vi "ATS_InputControl.vi"(7 "ID":i32, 9 "InputControl":T1 {"Range" items=["20mV", "40mV", "50mV", "80mV", "100mV", "200mV", "400mV", "500mV", "800mV", "1 V", "1.25 V", "2 V", "4 V", "5 V", "8 V", "10 V", "16 V", "20 V", "40 V", "HiFi"]}, 10 "Channel":T6, 11 "HandleIn":u32) -> (0 "Return Code":u32, 1 "OutputControl":T1 {"Range" items=["20mV", "40mV", "50mV", "80mV", "100mV", "200mV", "400mV", "500mV", "800mV", "1 V", "1.25 V", "2 V", "4 V", "5 V", "8 V", "10 V", "16 V", "20 V", "40 V", "HiFi"]}, 2 "Range_Value":dbl format="%.3f", 3 "HandleOut":u32)   [LabVIEW 2010]
doc: "_____AlazarTech, Scope_____\n\nConfigure an input channel for acquisition.\n\n- Channel\n- Coupling\n- Range\n- Impedance\n- Bandwidth (if applicable)"
uses:
  ATS_ctl/InputCtrl.ctl
  ATS_ctl/Coupling.ctl
  ATS_ctl/Range.ctl
  ATS_ctl/Impedance.ctl
  ATS_ctl/Bandwidth.ctl
  ATS_ctl/ATS_Channel.ctl
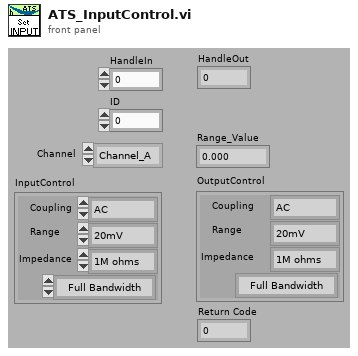
[diagram p1: front panel]
types:
  T1 = typedef "InputCtrl.ctl" = cluster{"Coupling":T2, "Range":T3, "Impedance":T4, "Bandwidth":T5}
  T2 = typedef "Coupling.ctl" = enum16{"AC", "DC"}
  T3 = typedef "Range.ctl" = u32
  T4 = typedef "Impedance.ctl" = enum16{"1M ohms", "50 ohms"}
  T5 = typedef "Bandwidth.ctl" = enum16{"Full Bandwidth", "Reduce Bandwidth"}
  T6 = typedef "ATS_Channel.ctl" = enum16{"Channel_A", "Channel_B", "Channel_C", "Channel_D"}
  T7 = typedef "ATS_Card_Spec.ctl" = cluster{"Name":string, "Rate":string[], "Range":string[], "RangeLim(50)":u32, "Bandwidth":bool}
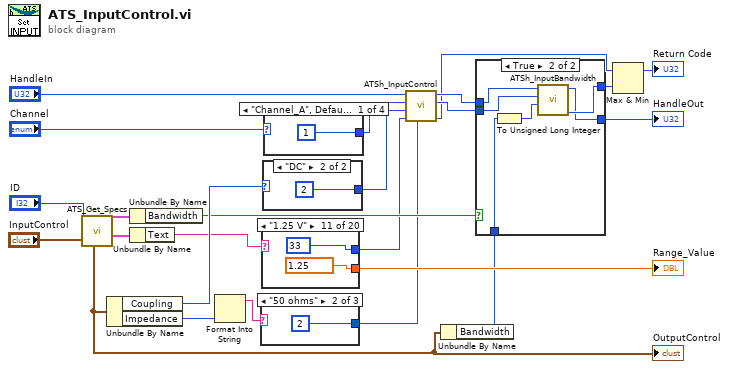
[diagram p0: block diagram]
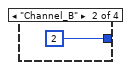
[diagram p2: hidden frame]
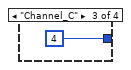
[diagram p3: hidden frame]
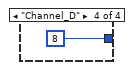
[diagram p4: hidden frame]
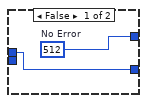
[diagram p5: hidden frame]
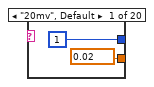
[diagram p6: hidden frame]
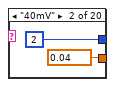
[diagram p7: hidden frame]
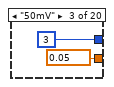
[diagram p8: hidden frame]
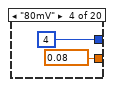
[diagram p9: hidden frame]
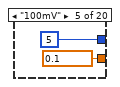
[diagram p10: hidden frame]
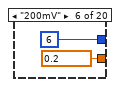
[diagram p11: hidden frame]
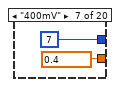
[diagram p12: hidden frame]
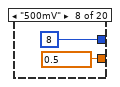
[diagram p13: hidden frame]
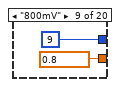
[diagram p14: hidden frame]
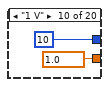
[diagram p15: hidden frame]
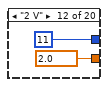
[diagram p16: hidden frame]
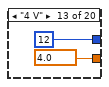
[diagram p17: hidden frame]
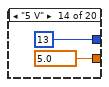
[diagram p18: hidden frame]
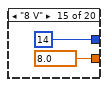
[diagram p19: hidden frame]
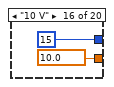
[diagram p20: hidden frame]
diagram:
  n1 = call "ATS_Get_Specs.vi"("InputControl"="InputControl", "ID"="ID") -> ("Range_Out"=w20:cluster{"Text":string, "Range":u32}, "Card_Spec"=w19:T7, "OutputControl"=w10:T1)  [unwired: 5 in, 2 out]
  "OutputControl" <- w10
  n2 = Unbundle By Name(w10) -> ("Coupling"=w24:T2, "Impedance"=w14:T4)
  n3 = Unbundle By Name(w19) -> ("Bandwidth"=w18:bool)
  n4 = Unbundle By Name(w20) -> ("Text"=w22:string)
  n5 = Format Into String(w14) -> (resulting string=w13:string)  [unwired: 3 in, 1 out]
  n6 = case shown="\"50 ohms\"" w13 {
    tunnel: [u32 1 ("Channel") u32 2 ("Channel") u32 8 ("Channel")] -> w5
    frame "1M ohms", Default {
    }
    frame "50 ohms" {
    }
    frame "300 ohms" {
    }
  }
  n7 = case shown="\"1.25 V\"" w22 {
    tunnel: [u32 1 ("Channel") u32 2 ("Channel") u32 3 ("Channel") u32 4 ("Channel") u32 5 ("Channel") u32 6 ("Channel") u32 7 ("Channel") u32 8 ("Channel") u32 9 ("Channel") u32 10 ("Channel") u32 33 ("Channel") u32 11 ("Channel") u32 12 ("Channel") u32 13 ("Channel") u32 14 ("Channel") u32 15 ("Channel") u32 18 ("Channel") u32 16 ("Channel") u32 17 ("Channel") u32 32 ("Channel")] -> w4
    tunnel: [0.02 ("Range_Value") 0.04 ("Range_Value") 0.05 ("Range_Value") 0.08 ("Range_Value") 0.1 ("Range_Value") 0.2 ("Range_Value") 0.4 ("Range_Value") 0.5 ("Range_Value") 0.8 ("Range_Value") 1.0 ("Range_Value") 1.25 ("Range_Value") 2.0 ("Range_Value") 4.0 ("Range_Value") 5.0 ("Range_Value") 8.0 ("Range_Value") 10.0 ("Range_Value") 16.0 ("Range_Value") 20.0 ("Range_Value") 40.0 ("Range_Value") 0.25 ("Range_Value")] -> w21
    frame "20mv", Default {
    }
    frame "40mV" {
    }
    frame "50mV" {
    }
    frame "80mV" {
    }
    frame "100mV" {
    }
    frame "200mV" {
    }
    frame "400mV" {
    }
    frame "500mV" {
    }
    frame "800mV" {
    }
    frame "1 V" {
    }
    frame "1.25 V" {
    }
    frame "2 V" {
    }
    frame "4 V" {
    }
    frame "5 V" {
    }
    frame "8 V" {
    }
    frame "10 V" {
    }
    frame "16 V" {
    }
    frame "20 V" {
    }
    frame "40 V" {
    }
    frame "HiFi" {
    }
  }
  "Range_Value" <- w21
  n8 = case shown="\"DC\"" w24 {
    tunnel: [u32 1 ("Channel") u32 2 ("Channel")] -> w3
    frame "AC", Default {
    }
    frame "DC" {
    }
  }
  n9 = case shown="\"Channel_A\", Default" "Channel" {
    tunnel: [u32 1 ("Channel") u32 2 ("Channel") u32 4 ("Channel") u32 8 ("Channel")] -> w1
    frame "Channel_A", Default {
    }
    frame "Channel_B" {
    }
    frame "Channel_C" {
    }
    frame "Channel_D" {
    }
  }
  n10 = call "ATSh_InputControl.vi"("Impedance"=w5, "InputRange"=w4, "Coupling"=w3, "Channel"=w1, "HandleIn"="HandleIn") -> ("Return"=w6:u32, "Channel_Out"=w7:u32, "Handle_Out"=w8:u32)  [unwired: 4 in]
  n11 = Unbundle By Name(w10) -> ("Bandwidth"=w11:T5)
  n12 = case shown="True" w18 {
    tunnel: [w74 w80] -> w16
    tunnel: w8 -> [w75 w76]
    tunnel: [w75 w79] -> w17
    tunnel: w7 -> [_ w77]
    tunnel: w11 -> [_ w81]
    frame False {
      w74 = u32 512  # No Error
    }
    frame True {
      n13 = To Unsigned Long Integer(number=w81) -> (unsigned 32bit integer=w78:u32)
      n14 = call "ATSh_InputBandwidth.vi"("Bandwidth"=w78, "Channel"=w77, "Handle"=w76) -> ("Return"=w80:u32, "Handle_out"=w79:u32)  [unwired: 7 in]
    }
  }
  "HandleOut" <- w17
  n15 = Max & Min(x=w6, y=w16) -> (max(x,y)=→"Return Code":u32)  [unwired: 1 out]
